vi "dc-potentional.vi"(2 "S":bool, 3 "C":bool, 4 "D":bool, 5 "R":bool) -> (0 "notQ":bool, 1 "Q":bool)   [LabVIEW 2013]
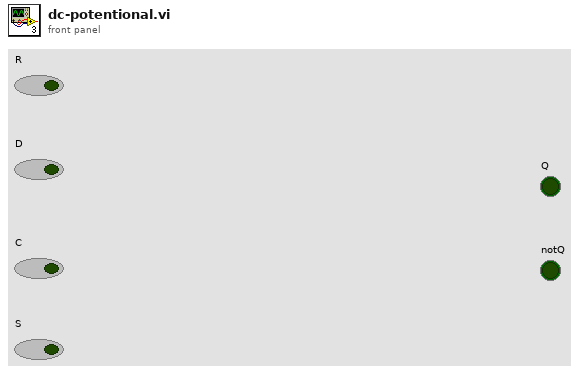
[diagram p1: front panel]
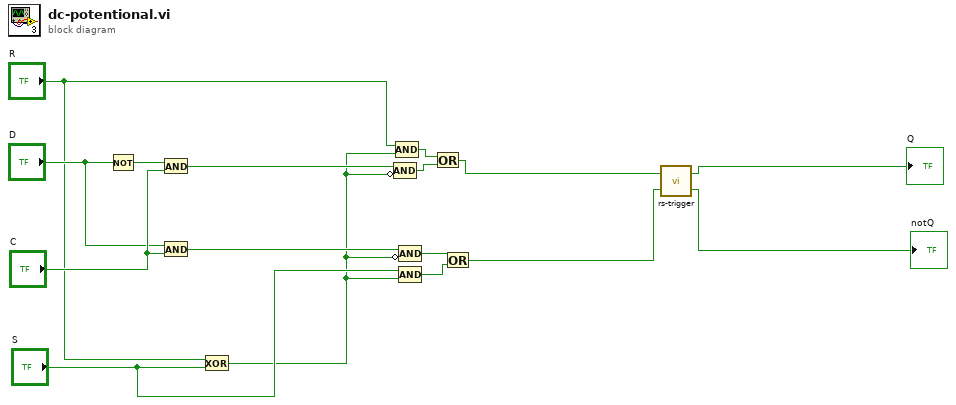
[diagram p0: block diagram]
diagram:
  n1 = Not(x="D") -> (.not. x?=w15:bool)
  n2 = And(x=w15, y="C") -> (x .and. y?=w9:bool)
  n3 = And(x="D", y="C") -> (x .and. y?=w8:bool)
  n4 = Exclusive Or(1:"S", 2:"R") -> (0:w7:bool)
  n5 = Compound Arithmetic op=AND(w9, invert w7) -> (w2:bool)
  n6 = Compound Arithmetic op=AND("R", w7) -> (w3:bool)
  n7 = Compound Arithmetic op=AND(w8, invert w7) -> (w6:bool)
  n8 = Compound Arithmetic op=AND("S", w7) -> (w5:bool)
  n9 = Or(x=w3, y=w2) -> (x .or. y?=w1:bool)
  n10 = Or(x=w6, y=w5) -> (x .or. y?=w4:bool)
  n11 = call "rs-trigger.vi"("S"=w4, "R"=w1) -> ("notQ"=→"notQ":bool, "Q"=→"Q":bool)
